vi "copy Complex Data to Array 2D.vi"(4 "error in (no error)":errorcluster, 7 "Complex Data":refnum<class "Complex Data.lvclass">) -> (0 "error out":errorcluster, 2 "Data Content":csg[][](array[numeric]), 3 "Complex Data out":refnum<class "Complex Data.lvclass">)   [LabVIEW 2017]
doc: "Copies the real and imaginary parts of the Complex Data object to 2D array of Float32."
uses:
  C:/Program Files/Thorlabs/SpectralRadar/LabVIEW/2012/user.lib/SpectralRadar.llb/Complex Data.lvclass
  C:/Program Files/Thorlabs/SpectralRadar/LabVIEW/2012/user.lib/SpectralRadar.llb/Data Property Int Selection.ctl
  C:/Program Files/Thorlabs/SpectralRadar/LabVIEW/2012/user.lib/SpectralRadar.llb/Data.lvclass
  SpectralRadar.dll
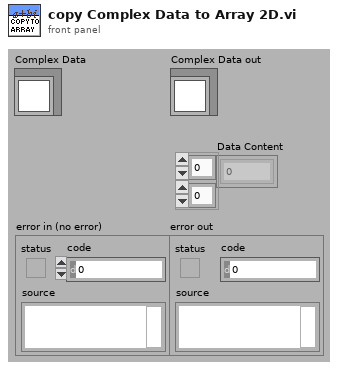
[diagram p1: front panel]
types:
  T1 = typedef "Data.lvclass/Data Property Int Selection.ctl" = enum16{"Dimensions", "Size 1", "Size 2", "Size 3", "Number of Data Points", "Data Size in Bytes", "Bytes per Pixel"}
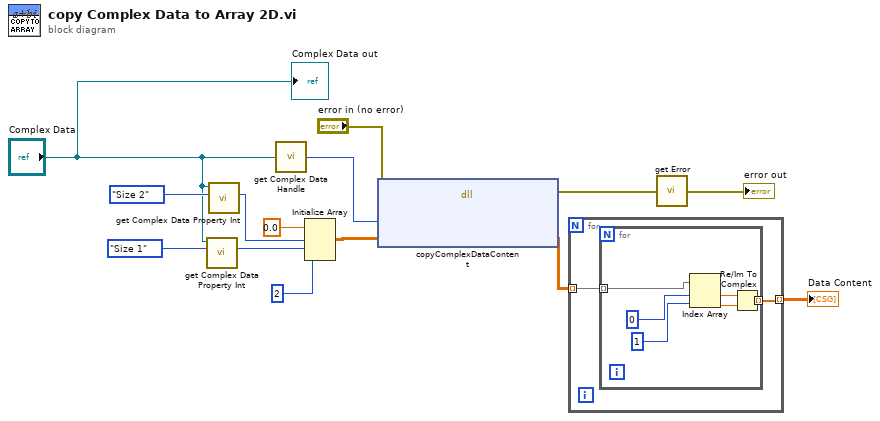
[diagram p0: block diagram]
diagram:
  n1 = call "get Complex Data Property Int.vi"("Data Property Selection"=Data_Property_Int_Selection."Size 1", "Complex Data"="Complex Data") -> ("Property Value"=w2:i32)  [unwired: 3 in, 2 out]
  n2 = call "get Complex Data Property Int.vi"("Data Property Selection"=Data_Property_Int_Selection."Size 2", "Complex Data"="Complex Data") -> ("Property Value"=w3:i32)  [unwired: 3 in, 2 out]
  n3 = call "get Complex Data Handle.vi"("Complex Data"="Complex Data") -> ("Handle"=w4:u64)
  n4 = Initialize Array(sgl 0.0 ("element"), w3, w2, 2 ("dimension size")) -> (w8:sgl[][][])
  n5 = dll-call lib="SpectralRadar.dll" fn="copyComplexDataContent"(error in="error in (no error)", "Data Handle"=w4, "Data Content"=w8) -> (error out=w12:errorcluster, "Data Content"=w7:sgl[][][])  [unwired: 4 in, 1 out]
  n6 = for {
    tunnel: w7 -> [w16] mode=indexing
    tunnel: [w15] -> w6 mode=indexing
    n7 = for {
      tunnel: w16 -> [w22] mode=indexing
      tunnel: [w17] -> w15 mode=indexing
      n8 = Index Array(array=w22, index #1=0 ("index"), index #2=1 ("index")) -> (element #1=w19:sgl, element #2=w18:sgl)
      n9 = Re/Im To Complex(1:w18, 2:w19) -> (0:w17:csg)
    }
  }
  "Data Content" <- w6
  n10 = call "get Error.vi"("error in (no error)"=w12) -> ("error out"=→"error out":errorcluster)
  "Complex Data out" <- "Complex Data"
